vi "test_CCDIsOpen.vi"(7 "Test should pass":bool=TRUE, 8 "error in":errorcluster, 9 "tear down connection":bool=TRUE, 10 "set-up a connection":bool=TRUE, 11 "device selection":enum16{"monochromator", "CCD", "SCD"}(ring)=enum."CCD") -> (0 "error out":errorcluster)   [LabVIEW 2023]
uses:
  <vilib>/addons/_JKI Toolkits/Caraya/classes/Test/Test.lvclass
  <vilib>/addons/_JKI Toolkits/Caraya/classes/Assert/Assert.lvclass
  <vilib>/addons/_JKI Toolkits/Caraya/classes/Assert/Assert Equal Value_Variant.vi
  Source/Classes/CCD/CCD.lvclass
  Source/Classes/SCD/SCD.lvclass
  Source/Classes/Mono/Monochromator.lvclass
  <vilib>/addons/_JKI Toolkits/Caraya/classes/Assert/Assert Not Error.vi
  C:/Users/grju/Desktop/AbgelegteDokumente/Kunden/Horiba/horiba-labview-sdk/Source/Classes/GenericDevice/GenericDevice.lvclass
  C:/Users/grju/Desktop/AbgelegteDokumente/Kunden/Horiba/horiba-labview-sdk/Source/Classes/CCD/CCD.lvclass
panel:
  # "Connector Pane"
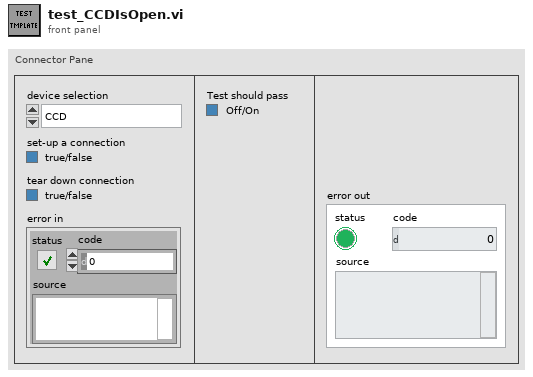
[diagram p1: front panel]
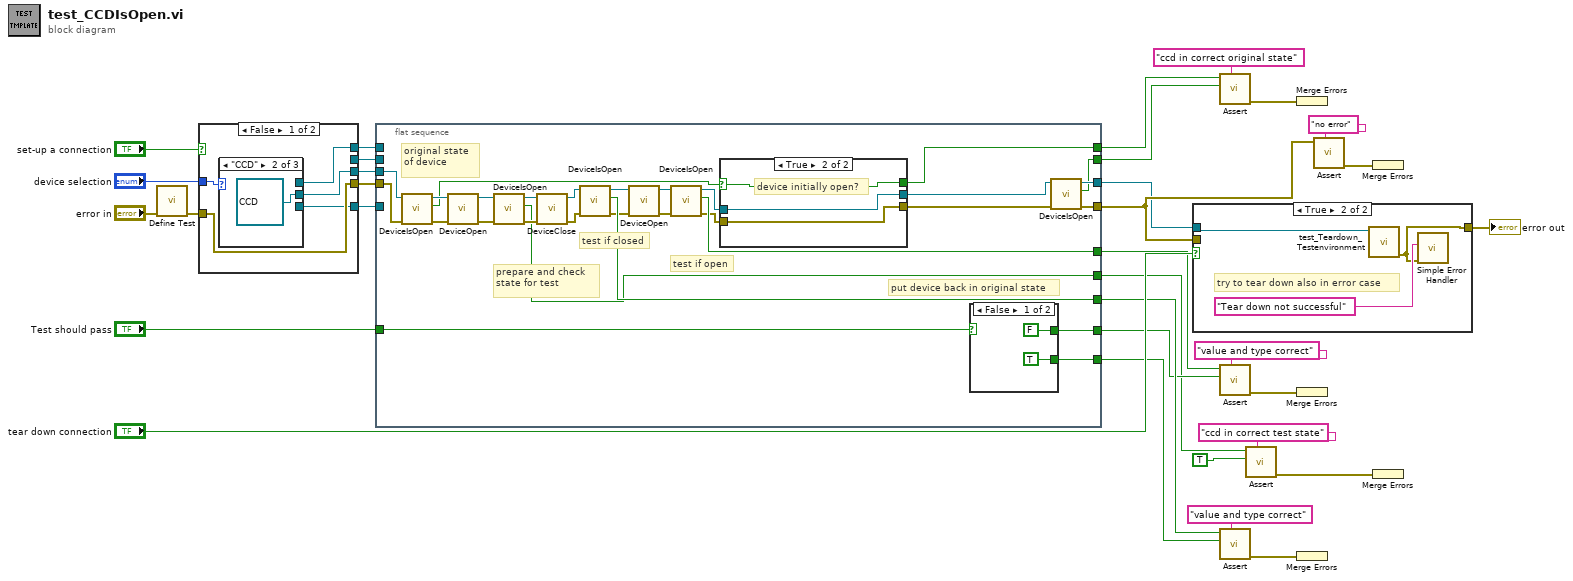
[diagram p0: block diagram]
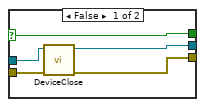
[diagram p2: hidden frame]
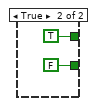
[diagram p3: hidden frame]
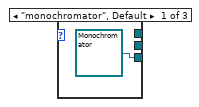
[diagram p5: hidden frame]
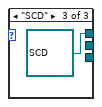
[diagram p6: hidden frame]
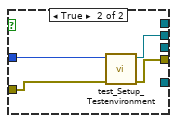
[diagram p7: hidden frame]
diagram:
  n1 = call <vilib>:"Define Test.vi"("error in (no error)"="error in") -> ("error out"=w24:errorcluster)  [unwired: 9 in, 1 out]
  n2 = case shown="False" "set-up a connection" {
    tunnel: w24 -> [w37 w44]
    tunnel: [w37 w43] -> w26
    tunnel: "device selection" -> [w36 w42]
    tunnel: [_ w41] -> w23
    tunnel: [w35 _] -> w22
    tunnel: [w34 _] -> w21
    tunnel: [w33 _] -> w20
    frame False {
      n3 = case shown="\"CCD\"" w36 {
        tunnel: [refnum<class "Monochromator.lvclass"> refnum ("Monochromator.lvclass") _ _] -> w35
        tunnel: [_ refnum<class "CCD.lvclass"> refnum ("CCD in") _] -> w34
        tunnel: [_ _ refnum<class "SCD.lvclass"> refnum ("SCD.lvclass")] -> w33
        frame "monochromator", Default {
        }
        frame "CCD" {
        }
        frame "SCD" {
        }
      }
    }
    frame True {
      n4 = call "test_Setup_Testenvironment.vi"("error in"=w44, "device selection"=w42) -> ("error out"=w43:errorcluster, "GenericDevice.lvclass"=w41:refnum<class "GenericDevice.lvclass">)  [unwired: 7 in, 1 out]
    }
  }
  n5 = flat-sequence {
    tunnel: w26 -> [w72]
    tunnel: w23 -> [_]
    tunnel: w22 -> [_]
    tunnel: w21 -> [w71]
    tunnel: w20 -> [_]
    tunnel: [w45] -> w14
    tunnel: "Test should pass" -> [w73]
    tunnel: [w49] -> w13
    tunnel: [w62] -> w12
    tunnel: [w61] -> w11
    tunnel: [w60] -> w10
    tunnel: [w59] -> w9
    tunnel: [w58] -> w6
    tunnel: [w51] -> w2
    tunnel: [w48] -> w1
    frame #0 {
      # "put device back in original state"
      # "test if open"
      # "test if closed"
      # "original state of device"
      # "prepare and check state for test"
      n6 = call-dynamic "DeviceIsOpen.vi"("error in (no error)"=w72, "CCD in"=w71) -> ("error out"=w63:errorcluster, "device is open?"=w57:bool, "CCD out"=w70:refnum<class "CCD.lvclass">)  [unwired: 6 in, 1 out]
      n7 = call-dynamic "DeviceOpen.vi"("error in (no error)"=w63, "CCD in"=w70) -> ("error out"=w64:errorcluster, "CCD out"=w69:refnum<class "CCD.lvclass">)  [unwired: 6 in, 2 out]
      n8 = call-dynamic "DeviceIsOpen.vi"("error in (no error)"=w64, "CCD in"=w69) -> ("error out"=w65:errorcluster, "device is open?"=w58:bool, "CCD out"=w68:refnum<class "CCD.lvclass">)  [unwired: 6 in, 1 out]
      n9 = call-dynamic "DeviceClose.vi"("error in (no error)"=w65, "CCD in"=w68) -> ("error out"=w66:errorcluster, "CCD out"=w67:refnum<class "CCD.lvclass">)  [unwired: 5 in, 3 out]
      n10 = call-dynamic "DeviceIsOpen.vi"("error in (no error)"=w66, "CCD in"=w67) -> ("error out"=w53:errorcluster, "device is open?"=w62:bool, "CCD out"=w55:refnum<class "CCD.lvclass">)  [unwired: 6 in, 1 out]
      n11 = call-dynamic "DeviceOpen.vi"("error in (no error)"=w53, "CCD in"=w55) -> ("error out"=w52:errorcluster, "CCD out"=w54:refnum<class "CCD.lvclass">)  [unwired: 6 in, 2 out]
      n12 = call-dynamic "DeviceIsOpen.vi"("error in (no error)"=w52, "CCD in"=w54) -> ("error out"=w47:errorcluster, "device is open?"=w60:bool, "CCD out"=w56:refnum<class "CCD.lvclass">)  [unwired: 6 in, 1 out]
      n13 = case shown="True" w57 {
        selector: w57 -> [w76 w79]
        tunnel: w56 -> [w78 w81]
        tunnel: [w77 w81] -> w50
        tunnel: [w76 w79] -> w51
        tunnel: w47 -> [w75 w80]
        tunnel: [w74 w80] -> w46
        frame False {
          n14 = call-dynamic "DeviceClose.vi"("error in (no error)"=w75, "CCD in"=w78) -> ("error out"=w74:errorcluster, "CCD out"=w77:refnum<class "CCD.lvclass">)  [unwired: 5 in, 3 out]
        }
        frame True {
          # "device initially open?"
        }
      }
      n15 = case shown="False" w73 {
        tunnel: [TRUE ("device is open?") FALSE ("device is open?")] -> w61
        tunnel: [FALSE ("device is open?") TRUE ("device is open?")] -> w59
        frame False {
        }
        frame True {
        }
      }
      n16 = call-dynamic "DeviceIsOpen.vi"("error in (no error)"=w46, "CCD in"=w50) -> ("error out"=w45:errorcluster, "device is open?"=w48:bool, "CCD out"=w49:refnum<class "CCD.lvclass">)  [unwired: 6 in, 1 out]
    }
  }
  n17 = case shown="True" "tear down connection" {
    tunnel: w13 -> [_ w88]
    tunnel: [w86 w87] -> w16
    tunnel: w14 -> [w86 _]
    frame False {
    }
    frame True {
      # "try to tear down also in error case"
      n18 = call "test_Teardown_Testenvironment.vi"("GenericDevice.lvclass"=w88) -> ("error out"=w87:errorcluster)  [unwired: 9 in, 1 out]
      n19 = call <vilib>:"Simple Error Handler.vi"("error source (\" \")"="Tear down not successful" ("error source (\" \")"), "error in (no error)"=w87) -> ()  [unwired: 3 in, 5 out]
    }
  }
  "error out" <- w16
  n20 = call-poly <vilib>:"Assert.vi"("Label"="ccd in correct original state" ("Label (VI Title)"), "Y"=w1, "X"=w2) -> ("error out"=w4:errorcluster)  [unwired: 7 in, 1 out]
  n21 = call-poly <vilib>:"Assert.vi"("Label"="value and type correct" ("Label (VI Title)"), "Y"=w9, "X"=w10) -> ("error out"=w28:errorcluster)  [unwired: 7 in, 1 out]
  n22 = call-poly <vilib>:"Assert.vi"("Label"="value and type correct" ("Label (VI Title)"), "Y"=w11, "X"=w12) -> ("error out"=w30:errorcluster)  [unwired: 7 in, 1 out]
  n23 = call-poly <vilib>:"Assert.vi"("Label"="ccd in correct test state" ("Label (VI Title)"), "Y"=TRUE ("device is open?"), "X"=w6) -> ("error out"=w8:errorcluster)  [unwired: 7 in, 1 out]
  n24 = Merge Errors(w4) -> ()  [unwired: 1 out]
  n25 = Merge Errors(w28) -> ()  [unwired: 1 out]
  n26 = Merge Errors(w30) -> ()  [unwired: 1 out]
  n27 = call-poly <vilib>:"Assert.vi"("Label"="no error" ("Label (VI Title)"), "Not Error?"=w14) -> ("error out"=w17:errorcluster)  [unwired: 8 in, 1 out]
  n28 = Merge Errors(w17) -> ()  [unwired: 1 out]
  n29 = Merge Errors(w8) -> ()  [unwired: 1 out]
